vi "Actor Core.vi"(8 "error in":errorcluster, 11 "LiveDatActor in":refnum<class "LiveDatActor.lvclass">) -> (0 "error out":errorcluster, 3 "Actor out":refnum<class "Actor.lvclass">)   [LabVIEW 2020, in "LiveDatActor.lvlib" / "LiveDatActor.lvclass"]
doc: "(<B>Filename</B>: Actor Framework.lvlib:Actor.lvclass:Actor Core.vi)\n\nReceives messages to the actor, reacts to them, and initiates any error handling that may shut the actor down.\n\nDescendant classes may override this VI to append parallel tasks for the actor to complete while it handles messages. Overrides use the Call Parent Method node."
uses:
  LiveDatActor.lvclass
  support/Actor Framework.lvlibp/1abvi3w/vi.lib/ActorFramework/Actor/Actor.lvclass
  LiveDatActor.lvclass/LiveDatActor.ctl
  support/UI_Actor.lvlibp/UI_Actor/UI_Actor.lvclass
panel:
  in  "Tree":string(tree)
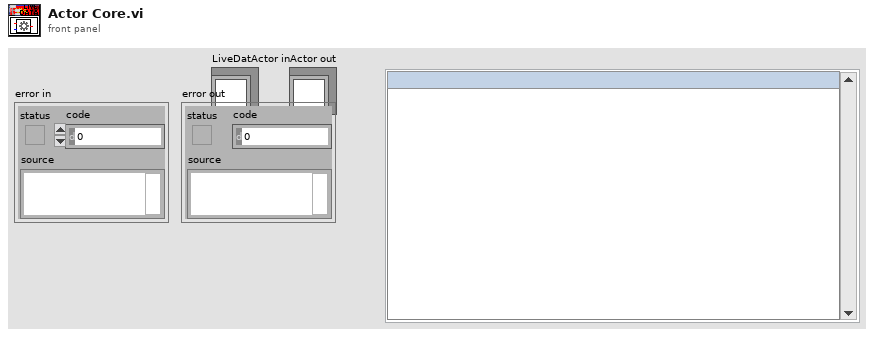
[diagram p1: front panel]
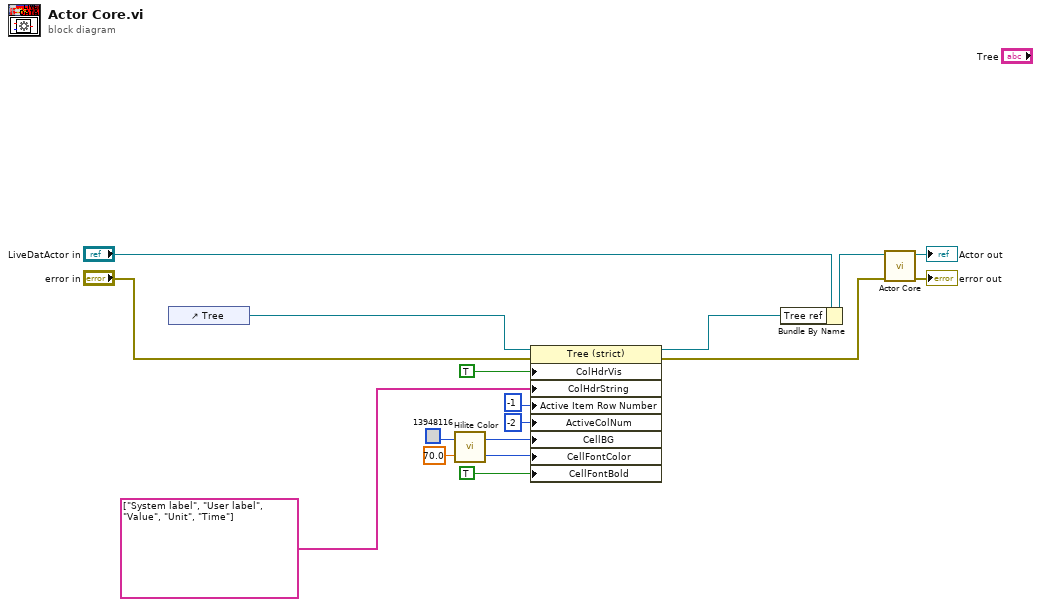
[diagram p0: block diagram]
diagram:
  n1 = control-ref of="Tree"() -> (w6:refnum<vi>)
  n2 = call <vilib>:"Hilite Color.vi"("Percentage(30)"=70.0, "Color In"=u32 13948116) -> ("Shadow"=w12:u32, "Hilite"=w13:u32)
  n3 = property class="Tree (strict)"(reference=w6, error in="error in", "ColHdrVis"=TRUE ("Visible Items:Column Headers Visible"), "ColHdrString"=string[] ["System label", "User label", "Value", "Unit", "Time"] ("Labels"), "Active Item Row Number"=-1 ("Active Cell:Active Column Number"), "ActiveColNum"=-2 ("Active Cell:Active Column Number"), "CellBG"=w13, "CellFontColor"=w12, "CellFontBold"=TRUE ("Visible Items:Column Headers Visible")) -> (reference out=w5:refnum<vi>, error out=w3:errorcluster)
  n4 = Bundle By Name(cluster="LiveDatActor in", "Tree ref"=w5) -> (w14:refnum<class "LiveDatActor.lvclass">)
  n5 = call-parent "Actor Core.vi"("error in"=w3, "UI_Actor in"=w14) -> ("error out"=→"error out":errorcluster, "Actor out"=→"Actor out":refnum<class "Actor.lvclass">)  [unwired: 8 in]
